vi "GetProperty.vi"(8 "error in (no error)":errorcluster, 10 "Property":string, 11 "CSSProperties in":refnum<class "CSSProperties.lvclass">) -> (0 "error out":errorcluster, 2 "Value":string, 3 "CSSProperties out":refnum<class "CSSProperties.lvclass">)   [LabVIEW 2019, in "CSSProperties.lvclass"]
uses:
  CSSProperties.lvclass
  CSSProperties.lvclass/CSSProperties.ctl
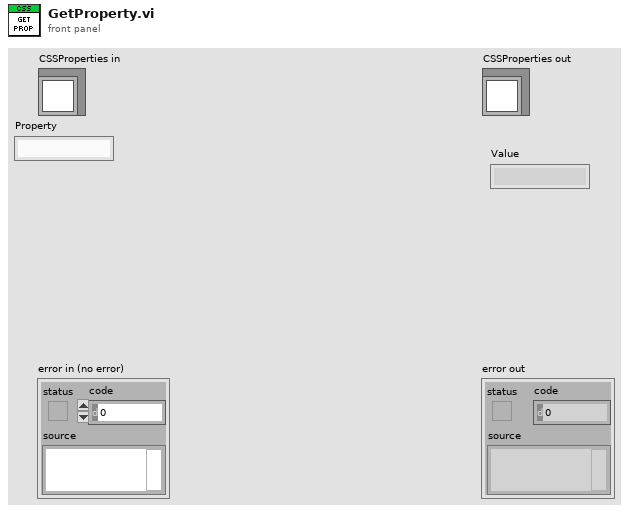
[diagram p1: front panel]
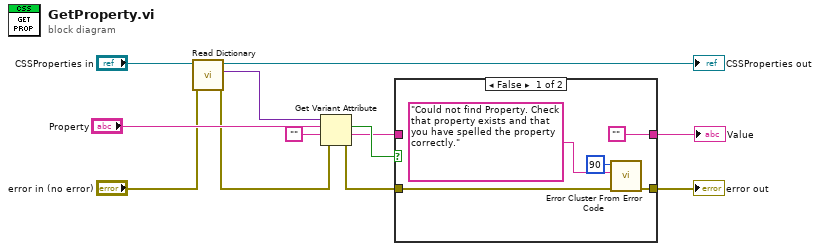
[diagram p0: block diagram]
diagram:
  n1 = call "Read Dictionary.vi"("error in (no error)"="error in (no error)", "CSSProperties in"="CSSProperties in") -> ("error out"=w2:errorcluster, "Dictionary"=w9:variant, "CSSProperties out"=→"CSSProperties out":refnum<class "CSSProperties.lvclass">)  [unwired: 7 in]
  n2 = Get Variant Attribute(Variant=w9, name="Property", default value (empty Variant)="", error in=w2) -> (found=w8:bool, value=w6:string, error out=w4:errorcluster)  [unwired: 1 out]
  n3 = case shown="False" w8 {
    tunnel: w4 -> [w15 w19]
    tunnel: [w16 w19] -> w7
    tunnel: w6 -> [_ w18]
    tunnel: ["" w18] -> w5
    frame False {
      n4 = call <vilib>:"Error Cluster From Error Code.vi"("error in (no error)"=w15, "error message (\"\")"="Could not find Property. Check that property exists and that you have spelled the property correctly." ("error message (\"\")"), "error code (0)"=90) -> ("error out"=w16:errorcluster)  [unwired: 6 in]
    }
    frame True {
    }
  }
  "error out" <- w7
  "Value" <- w5
